vi "Load and Validate_Extract Number.vi"(11 "String":string) -> (2 "Number Array":i32[](array[numeric]), 3 "Last number":i32)   [LabVIEW 2020, in "ProjectBuilder.lvlib"]
uses:
  ProjectBuilder.lvlib
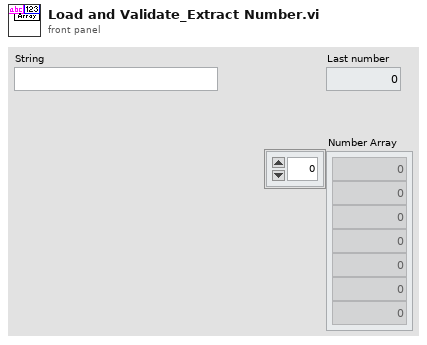
[diagram p1: front panel]
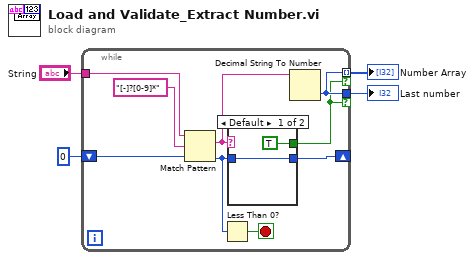
[diagram p0: block diagram]
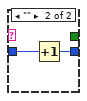
[diagram p2: hidden frame]
diagram:
  n1 = while {
    tunnel: [w6] -> w4 if=w5
    tunnel: "String" -> [w12]
    shift-right: [w9] -> _
    shift-left: 0 -> [w11]
    tunnel: [w6] -> w1 mode=indexing if=w5
    stop <- w7 stop-if-true
    n2 = Match Pattern(string=w12, regular expression="[-]?[0-9]*", offset (0)=w11) -> (match substring=w10:string, offset past match=w8:i32)  [unwired: 2 out]
    n3 = Less Than 0?(x=w8) -> (x < 0?=w7:bool)
    n4 = case shown="Default" w10 {
      tunnel: [w15 w16] -> w9
      tunnel: [TRUE _] -> w5
      tunnel: w8 -> [w15 w17]
      frame Default {
      }
      frame "" {
        n5 = Increment(x=w17) -> (x+1=w16:i32)
      }
    }
    n6 = Decimal String To Number(string=w10) -> (number=w6:i32)  [unwired: 2 in, 1 out]
  }
  "Last number" <- w4
  "Number Array" <- w1
